vi "Remove Duplicate Indexes.vi"(11 "Indexes In":i32[](array[numeric])) -> (3 "Indexes Out":i32[](array[numeric]))   [LabVIEW 2013]
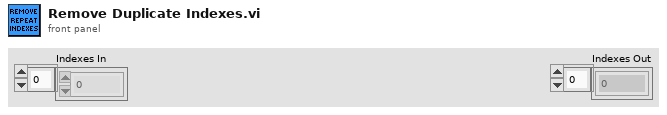
[diagram p1: front panel]
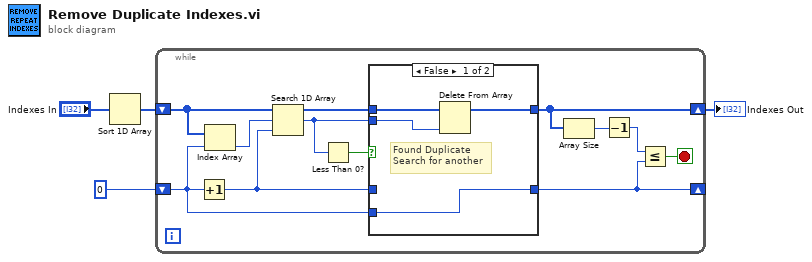
[diagram p0: block diagram]
diagram:
  n1 = Sort 1D Array(array="Indexes In") -> (sorted array=w3:i32[])
  n2 = while {
    shift-right: [w9] -> w1
    shift-left: w3 -> [w14]
    shift-right: [w8] -> _
    shift-left: 0 -> [w10]
    stop <- w7 stop-if-true
    n3 = Increment(x=w10) -> (x+1=w12:i32)
    n4 = Index Array(array=w14, index=w10) -> (element=w15:i32)
    n5 = Search 1D Array(1D array=w14, element=w15, start index (0)=w12) -> (index of element=w11:i32)
    n6 = Less Than 0?(x=w11) -> (x < 0?=w13:bool)
    n7 = case shown="False" w13 {
      tunnel: w14 -> [w19 w21]
      tunnel: [w18 w21] -> w9
      tunnel: w12 -> [_ w20]
      tunnel: [w16 w20] -> w8
      tunnel: w11 -> [w17 _]
      tunnel: w10 -> [w16 _]
      frame False {
        # "Found Duplicate\nSearch for another"
        n8 = Delete From Array(array=w19, index=w17) -> (array with subset deleted=w18:i32[])  [unwired: 1 in, 1 out]
      }
      frame True {
        # "No Duplicates"
      }
    }
    n9 = Array Size(array=w9) -> (size(s)=w6:i32)
    n10 = Decrement(x=w6) -> (x-1=w5:i32)
    n11 = Less Or Equal?(x=w5, y=w8) -> (x <= y?=w7:bool)
  }
  "Indexes Out" <- w1
